vi "Test_FormattedStringBinding_ValueOK.vi"(8 "error in (no error)":errorcluster, 11 "TestCase in":refnum<class "TestTransport.lvclass">) -> (0 "error out":errorcluster, 3 "TestCase out":refnum<class "TestTransport.lvclass">)   [LabVIEW 2017, in "TestTransport.lvclass"]
uses:
  TestTransport.lvclass
  FormattedStringBinding/FormattedStringBinding.lvclass/FormattedStringBinding.ctl
  FormattedStringBinding/FormattedStringBinding.lvclass
panel:
  out "String":string
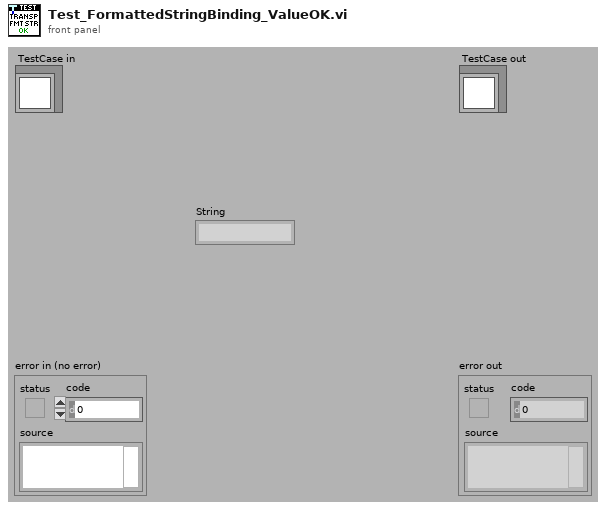
[diagram p1: front panel]
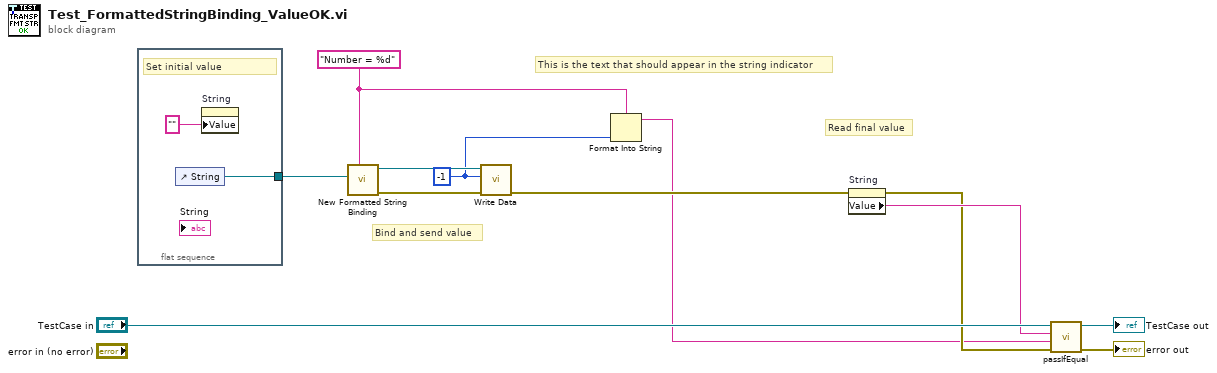
[diagram p0: block diagram]
diagram:
  w3 = "Number = %d" ("Format String")
  w2 = -1
  # "This is the text that should appear in the string indicator"
  # "Bind and send value"
  # "Read final value"
  n1 = flat-sequence {
    tunnel: [w14] -> w6
    frame #0 {
      # "Set initial value"
      n2 = control-ref of="String"() -> (w14:refnum<vi>)
      n3 = property on="String" class="Str"("Value"="" ("Boolean Text.Text")) -> ()  [unwired: 2 in, 2 out]
    }
  }
  n4 = call "New Formatted String Binding.vi"("Format String"=w3, "Str Refnum"=w6) -> ("error out"=w5:errorcluster, "FormattedStringBinding"=w8:refnum<class "FormattedStringBinding.lvclass">)  [unwired: 8 in]
  n5 = call-dynamic "Write Data.vi"("error in (no error)"=w5, "Value"=w2, "BooleanTextBinding in"=w8) -> ("error out"=w7:errorcluster)  [unwired: 7 in, 1 out]
  n6 = Format Into String(format string=w3, w2) -> (resulting string=w1:string)  [unwired: 2 in, 1 out]
  n7 = property on="String" class="Str"(error in=w7) -> (error out=w4:errorcluster, "Value"=w9:string)  [unwired: 1 in, 1 out]
  n8 = call-dynamic "passIfEqual.vi"("error in (no error)"=w4, "y"=w1, "x"=w9, "TestCase in"="TestCase in") -> ("error out"=→"error out":errorcluster, "TestCase out"=→"TestCase out":refnum<class "TestTransport.lvclass">)  [unwired: 6 in]
